vi "PH_Beamline.ProcCases.vi"(0 "i ref in":refnum<vi>, 1 "selector":string, 2 "Data":T1, 3 "call cluster":T2={"Object"="", "Selector"="", "CallType"=enum."synchronous", "Async Object"="", "Async Selector"="", "Data Descriptor"="", "Data"=[], "Error #"=0, "Expire"=0}, 5 "error in (no error)":errorcluster) -> (14 "i ref out":refnum<vi>, 17 "answer cluster":T2={"Object"="", "Selector"="", "CallType"=enum."synchronous", "Async Object"="", "Async Selector"="", "Data Descriptor"="", "Data"=[], "Error #"=0, "Expire"=0}, 19 "error out":errorcluster)   [LabVIEW 2014, in "PH_Beamline.lvlib"]
doc: "This method is called by a process from within the default case in the event loop. The methods of a class that are linked to events will be called from THIS method. Add your code here."
uses:
  PH_Beamline.lvlib
  CS_Core/CSSystem/CoreDefs/CoreDefs.call_type.ctl
  CS_Core/BaseProcess/BaseProcess.descriptor string definition.ctl
  CS_Core/CSSystem/CoreDefs/CoreDefs.rawDataType.ctl
  PH_Beamline_Chief/PH_Beamline_Chief.Settings.ctl
  PH_Basics/PH_StatusHandler/PH_StatusHandler.Status.ctl
  CS_Core/CSSystem/CoreLib/CoreLib.string 2 byte array.vi
  CS_Core/BaseProcess/BaseProcess.lvlib
  PH_Basics/PH_Common/PH_Common.lvlib
  CS_Core/CAEObj/CAEObj.lvlib
  CS_Core/CSSystem/CoreLib/CoreLib.lvlib
  PH_Basics/PH_StatusHandler/PH_StatusHandler.lvlib
  PH_BL-Master/PH_BL-Master.lvlib
  PH_Beamline_Chief/PH_Beamline_Chief.lvlib
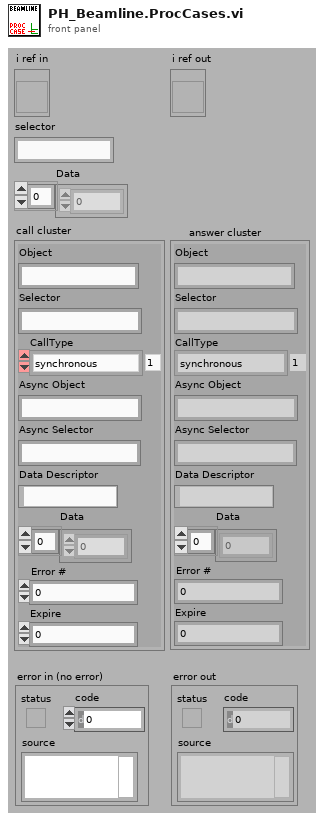
[diagram p1: front panel]
types:
  T1 = typedef "CoreDefs.rawDataType.ctl" = i8[]
  T2 = typedef "CoreDefs.call_type.ctl" = cluster{"Object":string, "Selector":string, "CallType":enum16{"simple", "synchronous", "asynchronous"}, "Async Object":string, "Async Selector":string, "Data Descriptor":T3, "Data":T1, "Error #":i32, "Expire":u32}
  T3 = typedef "BaseProcess.lvlib/BaseProcess.descriptor string definition.ctl" = string
  T4 = typedef "PH_Beamline_Chief.lvlib/PH_Beamline_Chief.Settings.ctl" = cluster{"PA Doublepass Mode":bool, "Compressor Vaccuum LB not relevant":bool, "Windowshutter TB2 not relevant":bool, "Windowshutter TB3 not relevant":bool}
  T5 = typedef "PH_BL-Master.lvlib/PH_BL-Master.i attribute.ctl" = cluster{"Remote controlled":bool, "Boolean Condition Service Subscriber":refnum<vi>[], "Picture Condition Service Subscriber":refnum<vi>[], "R2S":cluster{"GUI Ref":refnum<vi>, "State":bool}, "Vacua":cluster{"GUI Ref":refnum<vi>, "Limit":dbl, "Curr Value":dbl, "in range":bool}[], "O2 Inspection":cluster{"GUI Ref":refnum<vi>, "Concentration":dbl, "State":T6}[], "Boolean Status Service Subscriber":cluster{"GUI Ref":refnum<vi>, "Status":T6, "no Link?":bool, "Status Subscriber Class":T7}[], "Picture Status Service Subscriber":cluster{"GUI Ref":refnum<vi>, "Status":T6, "no Link?":bool, "Status Subscriber Class":T7}[], "6P 4Q Service Subscriber":cluster{"GUI Ref":refnum<vi>, "Selector":T8, "no Link?":bool}[], "Index of latest 6P 4Q changing Instance":i32, "Index of latest Picture Status changing Instance":i32, "Index of latest Boolean Status changing Instance":i32, "Vision ID on same Node":string, "Start Phase over?":bool, "GUI Ref Delete":refnum<vi>}
  T6 = typedef "PH_StatusHandler.lvlib/PH_StatusHandler.Status.ctl" = i16
  T7 = typedef "PH_BL-Master.lvlib/PH_BL-Master.Status Subscriber Class.ctl" = enum16{"unknown", "Switch", "BB", "6P Switch", "Switch GUI", "Switch and 6P State", "Force Sensor"}
  T8 = typedef "PH_4_Pos_Selector.lvlib/PH_4_Pos_Selector.Position Selector.ctl" = u16
  T9 = typedef "PH_Beamline.lvlib/PH_Beamline.i attribute.ctl" = cluster{"GUI Refs":cluster{"PA ok":refnum<vi>, "MA ok":refnum<vi>, "fs FE ok":refnum<vi>, "ns FE ok":refnum<vi>, "PA ED ok":refnum<vi>, "MAS ok":refnum<vi>, "Booster ok":refnum<vi>, "Mirrortower ok":refnum<vi>, "In.-Box ok":refnum<vi>, "Compressor ok":refnum<vi>, "Experiment LB ok":refnum<vi>, "Experiment LL ok":refnum<vi>, "PHELIX_Beckhoff_Watchdog":refnum<vi>, "Shutters closed":refnum<vi>, "uOPA ok":refnum<vi>, "Vacuum no shotcond Comp LB":refnum<vi>}, "Refs BL MA":refnum<vi>[], "Refs BL MA-IB":refnum<vi>[], "Refs BL fs":refnum<vi>[], "Refs BL PA ED":refnum<vi>[], "Refs BL MAS":refnum<vi>[], "Refs BL Boo":refnum<vi>[], "Refs BL ns":refnum<vi>[], "Refs BL Mirrortower":refnum<vi>[], "Refs BL Compressor":refnum<vi>[], "Refs BL Exp LB":refnum<vi>[], "Radiation Safety":cluster{"Exp Laserbay":cluster{"Ref Op Mode":refnum<vi>, "Ref Laserbay evacuated":refnum<vi>, "Tagname LB evacuated":string, "Shot Mode":T10, "Laserbay evacuated?":i32, "Tagname HV room locked":string, "HV room locked?":i32, "Ref HV room locked":refnum<vi>, "Tagname bridged?":string, "Ref Bridge":refnum<vi>, "I<1E18W/cm²":bool}, "Exp Laserlab":cluster{"Ref Op Mode":refnum<vi>, "Ref Laserlab evacuated":refnum<vi>, "Tagname LL evacuated":string, "Shot Mode":T10, "Laserlab evacuated?":i32, "Tagname bridged?":string, "Ref Bridge":refnum<vi>, "I<1E18W/cm²":bool}}, "Refs BL LL":refnum<vi>[], "PP Igni Heating GUI Refs":refnum<vi>[], "PP Igni Heating Tagnames ":string[], "Refs BL PA":cluster{"undelayed Line before Shutter":refnum<vi>[], "undelayed Line after Shutter":refnum<vi>[], "before Bypass":refnum<vi>[], "delayed Line before Shutter":refnum<vi>[], "delayed Line after Shutter":refnum<vi>[], "before Shutter Input":refnum<vi>[], "after Shutter Input":refnum<vi>[], "Bypass":refnum<vi>[], "before Shutter Exit":refnum<vi>[], "after Shutter Exit":refnum<vi>[], "to MA":refnum<vi>[], "to Lab":refnum<vi>[]}, "BL":cluster{"YLF_BL_Status":i32, "fs_BL_Status":i32, "fs_YLF_BL_Status":i32, "ns_BL_Status":i32, "PA_Input_BL_Status":i32, "PA_UnDelay_BL_Status":i32, "PA_Delay_BL_Status":i32, "PA_BL_Status":i32, "PA_Bypass_BL_Status":i32, "PA_Exit_BL_Status":i32, "PA_LL_BL_Status":i32, "LL_BL_Status":i32, "PA_MA_BL_Status":i32, "MA_Exit_BL_Status":i32, "MA_Z6_BL_Status":i32, "Z6_BL_Status":i32, "MA_LB_BL_Status":i32, "LB_TB2_BL_Status":i32, "PA_before_Bypass_BL_Status":i32, "LB_TB3_BL_Status":i32}, "State Subsystems":cluster{"PA":bool, "MA":bool, "ns FE":bool, "fs FE":bool, "PA ED":bool, "In.-Box":bool, "MAS":bool, "Booster":bool, "Mirrortower":bool, "Compressor":bool, "Experiment LB":bool, "Experiment LL":bool, "uOPA":bool}, "Status Subscriber Information":T11, "Refs BL uOPA":refnum<vi>[], "PA_Input_2_Beam_6PWpGUI not linked?":bool, "PA_Input_Delay_6PGUI not linked?":bool, "Settings":T4}
  T10 = typedef "PH_Beamline.lvlib/PH_Beamline.Operation Mode.ctl" = i32
  T11 = typedef "PH_Beamline.lvlib/PH_Beamline.Status Subscriber Information.ctl" = cluster{"fs Swich YLF":T12, "fs Exit Shutter":T12, "ns Exit Shutter":T12, "PA Input Shutter":T12, "PA PC WP":T12, "PA PC WP 2":T12, "PA Bypass In":T12, "PA Bypass Out":T12, "PA CH 1":T12, "PA delayed":T12, "PA non delayed":T12, "PA Exit Shutter":T12, "PA Switch Lab":T12, "PA Bridge CH Input MA":T12, "MA Diffusor IB":T12, "MA IB Ready":T12, "MA CH 1":T12, "MA CH 2":T12, "MA CH 3":T12, "MA CH 4":T12, "MA Shutter Align Cam":T12, "MA Position MM5":T12, "Calorimeter Switch":T12, "BL Z6 CH 9":T12, "BL Z6 Beamdump":T12, "BL Z6 Shutter":T12, "COS Sensitivity Switch":T12, "Exp LB Shutter":T12, "Exp LB TB 2":T12, "Exp LB TB 3":T12, "PA LL Input CH":T12, "PA LL Output CH":T12, "LL Comp Input Shutter":T12, "LL Comp Output Shutter":T12, "LL Comp FF Shutter":T12, "Exp LL Shutter":T12, "MA IM In IB":T12, "MA IM Out IB":T12, "MA DB In IB":T12, "MA DB Out IB":T12, "Exp LB Shutter Interlock":T12, "Exp LL Shutter Interlock":T12, "MM1 Force Sensor":T12}
  T12 = typedef "PH_BL-Master.lvlib/PH_BL-Master.Status Subscriber Information.ctl" = cluster{"Index of element":i32, "Attributeset":T13}
  T13 = typedef "PH_BL-Master.lvlib/PH_BL-Master.Attribute Set.ctl" = enum16{"Boolean Status Service Subscriber", "Picture Status Service Subscriber"}
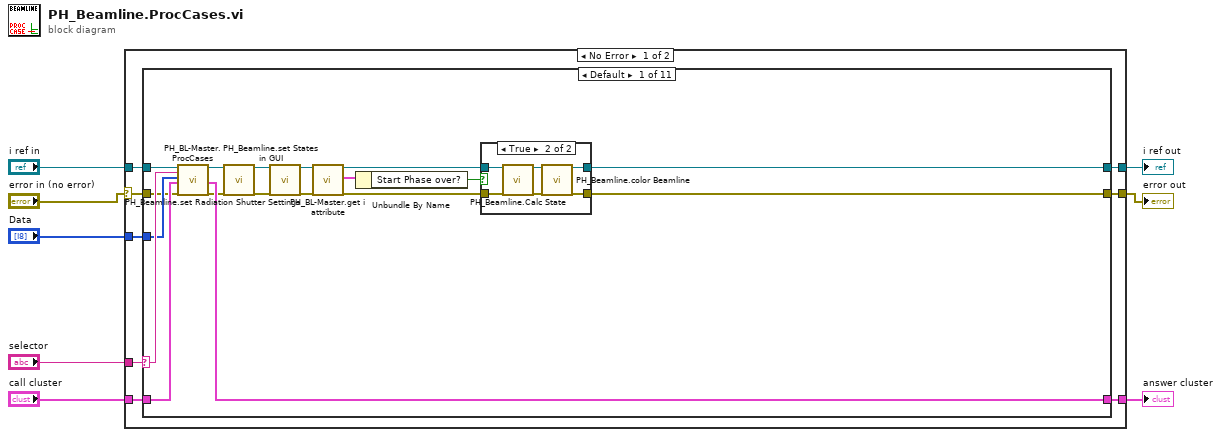
[diagram p0: block diagram]
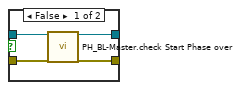
[diagram p2: hidden frame]
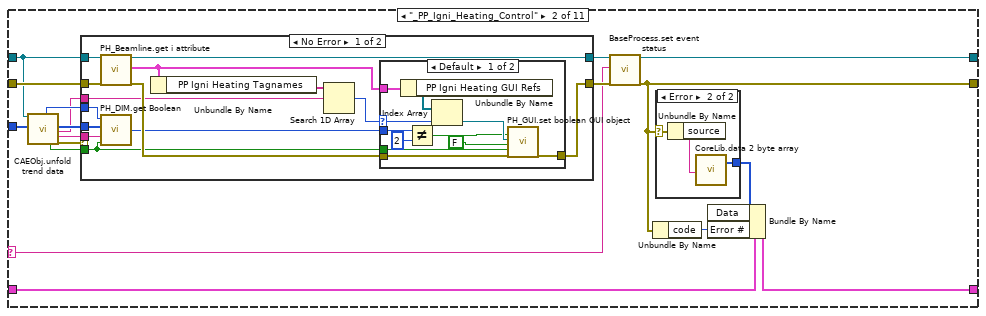
[diagram p3: hidden frame]
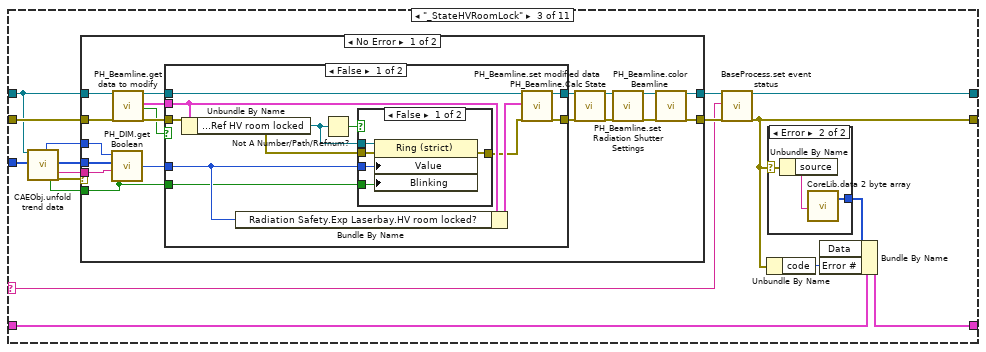
[diagram p7: hidden frame]
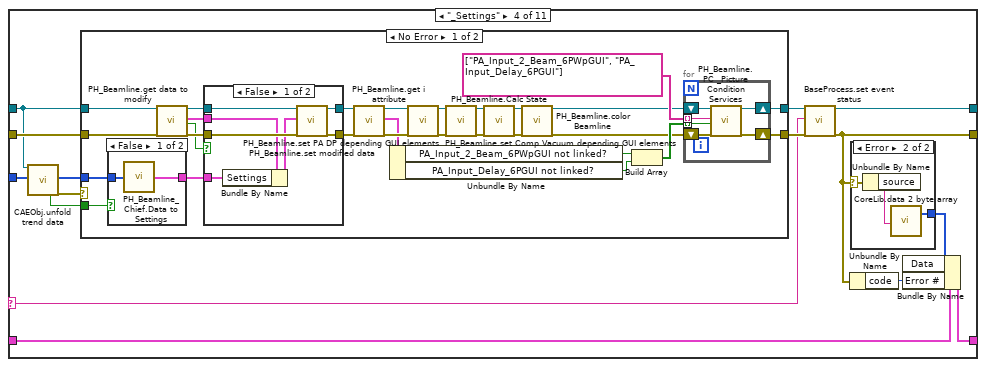
[diagram p12: hidden frame]
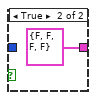
[diagram p14: hidden frame]
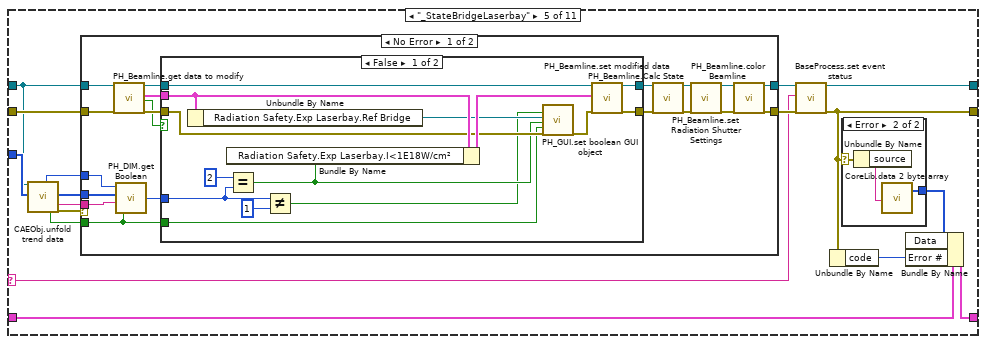
[diagram p17: hidden frame]
diagram:
  n1 = case shown="No Error" "error in (no error)" {
    selector: "error in (no error)" -> [w9 w487]
    tunnel: "selector" -> [w16 _]
    tunnel: [w15 w486] -> w7
    tunnel: "call cluster" -> [w14 w486]
    tunnel: "i ref in" -> [w13 w488]
    tunnel: [w12 w488] -> w4
    tunnel: [w11 w487] -> w3
    tunnel: "Data" -> [w10 _]
    frame No Error {
      n2 = case shown="Default" w16 {
        selector: w16 -> [w32 w47 w96 w156 w222 w279 w338 w371 w409 w445 w479]
        tunnel: w13 -> [w19 w60 w108 w166 w234 w291 w347 w383 w421 w454 w473]
        tunnel: [w31 w48 w97 w157 w223 w280 w339 w372 w410 w448 w478] -> w12
        tunnel: w14 -> [w33 w46 w95 w155 w221 w278 w337 w370 w408 w446 w476]
        tunnel: [w34 w45 w94 w154 w220 w277 w336 w369 w407 w444 w475] -> w15
        tunnel: w9 -> [w20 w62 w110 w168 w236 w293 w349 w385 w423 w457 w474]
        tunnel: [w30 w49 w98 w158 w224 w281 w340 w373 w411 w447 w477] -> w11
        tunnel: w10 -> [w29 w61 w109 w167 w235 w292 w348 w384 w422 w456 _]
        frame Default {
          n3 = call "PH_BL-Master.ProcCases.vi"("i ref in"=w19, "selector"=w32, "Data"=w29, "call cluster"=w33, "error in (no error)"=w20) -> ("i ref out"=w17:refnum<vi>, "answer cluster"=w34:T2, "error out"=w18:errorcluster)  [unwired: 12 in]
          n4 = call "PH_Beamline.set States in GUI.vi"("i ref in"=w17, "error in"=w18) -> ("i ref out"=w21:refnum<vi>, "error out"=w22:errorcluster)  [unwired: 16 in]
          n5 = call "PH_Beamline.set Radiation Shutter Settings.vi"("i ref in"=w21, "error in"=w22) -> ("i ref out"=w26:refnum<vi>, "error out"=w28:errorcluster)  [unwired: 16 in]
          n6 = call "PH_BL-Master.get i attribute.vi"("i ref in"=w26, "error in (no error)"=w28) -> ("i ref out"=w25:refnum<vi>, "i attribute"=w24:T5, "error out"=w27:errorcluster)  [unwired: 15 in]
          n7 = Unbundle By Name(w24) -> ("Start Phase over?"=w23:bool)
          n8 = case shown="True" w23 {
            tunnel: [w37 w44] -> w31
            tunnel: [w35 w43] -> w30
            tunnel: w27 -> [w36 w40]
            tunnel: w25 -> [w38 w39]
            frame False {
              n9 = call "PH_BL-Master.check Start Phase over.vi"("VI in"=w38, "error in (no error)"=w36) -> ("VI out"=w37:refnum<vi>, "error out"=w35:errorcluster)  [unwired: 16 in]
            }
            frame True {
              n10 = call "PH_Beamline.Calc State.vi"("i ref in"=w39, "error in (no error)"=w40) -> ("i ref out"=w42:refnum<vi>, "error out"=w41:errorcluster)  [unwired: 16 in]
              n11 = call "PH_Beamline.color Beamline.vi"("i ref in"=w42, "error in (no error)"=w41) -> ("i ref out"=w44:refnum<vi>, "error out"=w43:errorcluster)  [unwired: 16 in]
            }
          }
        }
        frame "_PP_Igni_Heating_Control" {
          n12 = call "CAEObj.unfold trend data.vi"("i ref in"=w60, "raw trend data"=w61) -> ("quality"=w58:i32, "no link"=w57:bool, "data"=w56:i8[], "serviceName"=w54:string, "typeDescriptor"=w55:string, "error out"=w59:errorcluster)  [unwired: 9 in, 3 out]
          n13 = case shown="No Error" w59 {
            tunnel: [w70 w93] -> w51
            tunnel: w60 -> [w74 w93]
            tunnel: w62 -> [w73 w92]
            tunnel: [w69 w92] -> w50
            tunnel: w58 -> [w77 _]
            tunnel: w57 -> [w66 _]
            tunnel: w56 -> [w76 _]
            tunnel: w55 -> [w75 _]
            tunnel: w54 -> [w78 _]
            frame No Error {
              n14 = call "PH_Beamline.get i attribute.vi"("i ref in"=w74, "error in (no error)"=w73) -> ("i ref out"=w70:refnum<vi>, "i attribute"=w68:T9, "error out"=w79:errorcluster)  [unwired: 15 in]
              n15 = call "PH_DIM.get Boolean.vi"("no link"=w66, "typeDescriptor"=w75, "data"=w76, "quality"=w77) -> ("Value"=w67:i32)
              n16 = Unbundle By Name(w68) -> ("PP Igni Heating Tagnames"=w71:string[])
              n17 = Search 1D Array(1D array=w71, element=w78) -> (index of element=w72:i32)  [unwired: 1 in]
              n18 = case shown="Default" w72 {
                selector: w72 -> [w86 _]
                tunnel: w68 -> [w88 _]
                tunnel: w79 -> [w90 w91]
                tunnel: [w89 w91] -> w69
                tunnel: w67 -> [w84 _]
                tunnel: w66 -> [w81 _]
                frame Default {
                  n19 = Unbundle By Name(w88) -> ("PP Igni Heating GUI Refs"=w87:refnum<vi>[])
                  n20 = Not Equal?(x=w84, y=2) -> (x != y?=w82:bool)
                  n21 = Index Array(array=w87, index=w86) -> (element=w85:refnum<vi>)
                  n22 = call "PH_GUI.set boolean GUI object.vi"("Visible (true)"=w82, "Boolean Knob GUI Ref"=w85, "Value"=FALSE, "Blinking? (false)"=w81, "error in (no error)"=w90) -> ("error out"=w89:errorcluster)  [unwired: 14 in]
                }
                frame -1 {
                }
              }
            }
            frame Error {
            }
          }
          n23 = call "BaseProcess.set event status.vi"("i ref in"=w51, "EventStatus"=w47, "error in (no error)"=w50) -> ("i ref out"=w48:refnum<vi>, "error out"=w49:errorcluster)  [unwired: 14 in, 1 out]
          n24 = Unbundle By Name(w49) -> ("code"=w53:i32)
          n25 = case shown="Error" w49 {
            selector: w49 -> [_ w65]
            tunnel: [_ w63] -> w52
            frame No Error {
            }
            frame Error {
              n26 = Unbundle By Name(w65) -> ("source"=w64:string)
              n27 = call-poly "CoreLib.data 2 byte array.vi"("string"=w64) -> ("byteArray out"=w63:T1)  [unwired: 18 in]
            }
          }
          n28 = Bundle By Name(cluster=w46, "Data"=w52, "Error #"=w53) -> (w45:T2)
        }
        frame "_StateHVRoomLock" {
          n29 = call "CAEObj.unfold trend data.vi"("i ref in"=w108, "raw trend data"=w109) -> ("quality"=w106:i32, "no link"=w105:bool, "data"=w104:i8[], "typeDescriptor"=w103:string, "error out"=w107:errorcluster)  [unwired: 9 in, 4 out]
          n30 = case shown="No Error" w107 {
            tunnel: [w119 w153] -> w100
            tunnel: w108 -> [w129 w153]
            tunnel: w110 -> [w128 w152]
            tunnel: [w115 w152] -> w99
            tunnel: w106 -> [w132 _]
            tunnel: w105 -> [w124 _]
            tunnel: w104 -> [w131 _]
            tunnel: w103 -> [w130 _]
            frame No Error {
              n31 = call "PH_DIM.get Boolean.vi"("no link"=w124, "typeDescriptor"=w130, "data"=w131, "quality"=w132) -> ("Value"=w125:i32)
              n32 = call "PH_Beamline.get data to modify.vi"("i ref in"=w129, "error in (no error)"=w128) -> ("i ref out"=w127:refnum<vi>, "i attribute"=w126:T9, "timed out"=w122:bool, "error out"=w123:errorcluster)  [unwired: 14 in]
              n33 = case shown="False" w122 {
                tunnel: w127 -> [w143 w151]
                tunnel: [w142 w151] -> w118
                tunnel: [w141 w150] -> w114
                tunnel: w126 -> [w140 _]
                tunnel: w125 -> [w137 _]
                tunnel: w124 -> [w136 _]
                tunnel: w123 -> [w134 w150]
                frame False {
                  n34 = Unbundle By Name(w140) -> ("Radiation Safety.Exp Laserbay.Ref HV room locked"=w135:refnum<vi>)
                  n35 = Bundle By Name(cluster=w140, "Radiation Safety.Exp Laserbay.HV room locked?"=w137) -> (w139:T9)
                  n36 = Not A Number/Path/Refnum?(number/path/refnum=w135) -> (NaN/Path/Refnum?=w138:bool)
                  n37 = case shown="False" w138 {
                    tunnel: w134 -> [w148 w149]
                    tunnel: [w147 w149] -> w133
                    tunnel: w135 -> [w146 _]
                    tunnel: w137 -> [w145 _]
                    tunnel: w136 -> [w144 _]
                    frame False {
                      n38 = property class="Ring (strict)"(reference=w146, error in=w148, "Value"=w145, "Blinking"=w144) -> (error out=w147:errorcluster)  [unwired: 1 out]
                    }
                    frame True {
                    }
                  }
                  n39 = call "PH_Beamline.set modified data.vi"("i ref in"=w143, "i attribute"=w139, "error in (no error)"=w133) -> ("i ref out"=w142:refnum<vi>, "error out"=w141:errorcluster)  [unwired: 15 in]
                }
                frame True {
                }
              }
              n40 = call "PH_Beamline.Calc State.vi"("i ref in"=w118, "error in (no error)"=w114) -> ("i ref out"=w121:refnum<vi>, "error out"=w117:errorcluster)  [unwired: 16 in]
              n41 = call "PH_Beamline.set Radiation Shutter Settings.vi"("i ref in"=w121, "error in"=w117) -> ("i ref out"=w120:refnum<vi>, "error out"=w116:errorcluster)  [unwired: 16 in]
              n42 = call "PH_Beamline.color Beamline.vi"("i ref in"=w120, "error in (no error)"=w116) -> ("i ref out"=w119:refnum<vi>, "error out"=w115:errorcluster)  [unwired: 16 in]
            }
            frame Error {
            }
          }
          n43 = call "BaseProcess.set event status.vi"("i ref in"=w100, "EventStatus"=w96, "error in (no error)"=w99) -> ("i ref out"=w97:refnum<vi>, "error out"=w98:errorcluster)  [unwired: 14 in, 1 out]
          n44 = Unbundle By Name(w98) -> ("code"=w102:i32)
          n45 = case shown="Error" w98 {
            selector: w98 -> [_ w113]
            tunnel: [_ w111] -> w101
            frame No Error {
            }
            frame Error {
              n46 = Unbundle By Name(w113) -> ("source"=w112:string)
              n47 = call-poly "CoreLib.data 2 byte array.vi"("string"=w112) -> ("byteArray out"=w111:T1)  [unwired: 18 in]
            }
          }
          n48 = Bundle By Name(cluster=w95, "Data"=w101, "Error #"=w102) -> (w94:T2)
        }
        frame "_Settings" {
          n49 = call "CAEObj.unfold trend data.vi"("i ref in"=w166, "raw trend data"=w167) -> ("no link"=w164:bool, "data"=w163:i8[], "error out"=w165:errorcluster)  [unwired: 9 in, 6 out]
          n50 = case shown="No Error" w165 {
            tunnel: [w173 w219] -> w160
            tunnel: w166 -> [w199 w219]
            tunnel: w168 -> [w198 w218]
            tunnel: [w172 w218] -> w159
            tunnel: w164 -> [w192 _]
            tunnel: w163 -> [w193 _]
            frame No Error {
              n51 = case shown="False" w192 {
                tunnel: w193 -> [w207 _]
                tunnel: [w206 T4 {"PA Doublepass Mode"=FALSE, "Compressor Vaccuum LB not relevant"=FALSE, "Windowshutter TB2 not relevant"=FALSE, "Windowshutter TB3 not relevant"=FALSE} ("Settings")] -> w191
                frame False {
                  n52 = call "PH_Beamline_Chief.Data to Settings.vi"("data"=w207) -> ("Settings"=w206:T4)
                }
                frame True {
                }
              }
              n53 = call "PH_Beamline.get data to modify.vi"("i ref in"=w199, "error in (no error)"=w198) -> ("i ref out"=w197:refnum<vi>, "i attribute"=w196:T9, "timed out"=w194:bool, "error out"=w195:errorcluster)  [unwired: 14 in]
              n54 = case shown="False" w194 {
                tunnel: w197 -> [w215 w217]
                tunnel: [w210 w217] -> w182
                tunnel: [w211 w216] -> w184
                tunnel: w196 -> [w212 _]
                tunnel: w195 -> [w214 w216]
                tunnel: w191 -> [w209 _]
                frame False {
                  n55 = Bundle By Name(cluster=w212, "Settings"=w209) -> (w213:T9)
                  n56 = call "PH_Beamline.set modified data.vi"("i ref in"=w215, "i attribute"=w213, "error in (no error)"=w214) -> ("i ref out"=w210:refnum<vi>, "error out"=w211:errorcluster)  [unwired: 15 in]
                }
                frame True {
                }
              }
              n57 = call "PH_Beamline.get i attribute.vi"("i ref in"=w182, "error in (no error)"=w184) -> ("i ref out"=w181:refnum<vi>, "i attribute"=w176:T9, "error out"=w183:errorcluster)  [unwired: 15 in]
              n58 = Unbundle By Name(w176) -> ("PA_Input_2_Beam_6PWpGUI not linked?"=w177:bool, "PA_Input_Delay_6PGUI not linked?"=w178:bool)
              n59 = call "PH_Beamline.set PA DP depending GUI elements.vi"("VI in"=w181, "error in (no error)"=w183) -> ("VI out"=w190:refnum<vi>, "error out"=w189:errorcluster)  [unwired: 16 in]
              n60 = call "PH_Beamline.set Comp Vacuum depending GUI elements.vi"("VI in"=w190, "error in (no error)"=w189) -> ("VI out"=w188:refnum<vi>, "error out"=w186:errorcluster)  [unwired: 16 in]
              n61 = call "PH_Beamline.Calc State.vi"("i ref in"=w188, "error in (no error)"=w186) -> ("i ref out"=w187:refnum<vi>, "error out"=w185:errorcluster)  [unwired: 16 in]
              n62 = call "PH_Beamline.color Beamline.vi"("i ref in"=w187, "error in (no error)"=w185) -> ("i ref out"=w175:refnum<vi>, "error out"=w174:errorcluster)  [unwired: 16 in]
              n63 = Build Array(w177, w178) -> (w179:bool[])
              n64 = for {
                tunnel: w179 -> [w201] mode=indexing
                tunnel: string[] ["PA_Input_2_Beam_6PWpGUI", "PA_Input_Delay_6PGUI"] -> [w200] mode=indexing
                shift-right: [w204] -> w173
                shift-left: w175 -> [w205]
                shift-right: [w202] -> w172
                shift-left: w174 -> [w203]
                n65 = call "PH_Beamline.PC _Picture Condition Services.vi"("i ref in"=w205, "Instancename"=w200, "No Link?"=w201, "error IO"=w203) -> ("i ref out"=w204:refnum<vi>, "error out"=w202:errorcluster)  [unwired: 14 in]
              }
            }
            frame Error {
            }
          }
          n66 = call "BaseProcess.set event status.vi"("i ref in"=w160, "EventStatus"=w156, "error in (no error)"=w159) -> ("i ref out"=w157:refnum<vi>, "error out"=w158:errorcluster)  [unwired: 14 in, 1 out]
          n67 = Unbundle By Name(w158) -> ("code"=w162:i32)
          n68 = case shown="Error" w158 {
            selector: w158 -> [_ w171]
            tunnel: [_ w169] -> w161
            frame No Error {
            }
            frame Error {
              n69 = Unbundle By Name(w171) -> ("source"=w170:string)
              n70 = call-poly "CoreLib.data 2 byte array.vi"("string"=w170) -> ("byteArray out"=w169:T1)  [unwired: 18 in]
            }
          }
          n71 = Bundle By Name(cluster=w155, "Data"=w161, "Error #"=w162) -> (w154:T2)
        }
        frame "_StateBridgeLaserbay" {
          n72 = call "CAEObj.unfold trend data.vi"("i ref in"=w234, "raw trend data"=w235) -> ("quality"=w232:i32, "no link"=w231:bool, "data"=w230:i8[], "typeDescriptor"=w229:string, "error out"=w233:errorcluster)  [unwired: 9 in, 4 out]
          n73 = case shown="No Error" w233 {
            tunnel: [w245 w276] -> w226
            tunnel: w234 -> [w255 w276]
            tunnel: w236 -> [w254 w275]
            tunnel: [w241 w275] -> w225
            tunnel: w232 -> [w258 _]
            tunnel: w231 -> [w250 _]
            tunnel: w230 -> [w257 _]
            tunnel: w229 -> [w256 _]
            frame No Error {
              n74 = call "PH_Beamline.get data to modify.vi"("i ref in"=w255, "error in (no error)"=w254) -> ("i ref out"=w253:refnum<vi>, "i attribute"=w252:T9, "timed out"=w248:bool, "error out"=w249:errorcluster)  [unwired: 14 in]
              n75 = call "PH_DIM.get Boolean.vi"("no link"=w250, "typeDescriptor"=w256, "data"=w257, "quality"=w258) -> ("Value"=w251:i32)
              n76 = case shown="False" w248 {
                tunnel: w253 -> [w272 w274]
                tunnel: [w271 w274] -> w244
                tunnel: [w270 w273] -> w240
                tunnel: w252 -> [w269 _]
                tunnel: w251 -> [w261 _]
                tunnel: w250 -> [w264 _]
                tunnel: w249 -> [w267 w273]
                frame False {
                  n77 = Unbundle By Name(w269) -> ("Radiation Safety.Exp Laserbay.Ref Bridge"=w265:refnum<vi>)
                  n78 = Equal?(x=2, y=w261) -> (x = y?=w262:bool)
                  n79 = Bundle By Name(cluster=w269, "Radiation Safety.Exp Laserbay.I<1E18W/cm²"=w262) -> (w268:T9)
                  n80 = Not Equal?(x=w261, y=1) -> (x != y?=w259:bool)
                  n81 = call "PH_GUI.set boolean GUI object.vi"("Visible (true)"=w259, "Boolean Knob GUI Ref"=w265, "Value"=w262, "Blinking? (false)"=w264, "error in (no error)"=w267) -> ("error out"=w266:errorcluster)  [unwired: 14 in]
                  n82 = call "PH_Beamline.set modified data.vi"("i ref in"=w272, "i attribute"=w268, "error in (no error)"=w266) -> ("i ref out"=w271:refnum<vi>, "error out"=w270:errorcluster)  [unwired: 15 in]
                }
                frame True {
                }
              }
              n83 = call "PH_Beamline.Calc State.vi"("i ref in"=w244, "error in (no error)"=w240) -> ("i ref out"=w247:refnum<vi>, "error out"=w243:errorcluster)  [unwired: 16 in]
              n84 = call "PH_Beamline.set Radiation Shutter Settings.vi"("i ref in"=w247, "error in"=w243) -> ("i ref out"=w246:refnum<vi>, "error out"=w242:errorcluster)  [unwired: 16 in]
              n85 = call "PH_Beamline.color Beamline.vi"("i ref in"=w246, "error in (no error)"=w242) -> ("i ref out"=w245:refnum<vi>, "error out"=w241:errorcluster)  [unwired: 16 in]
            }
            frame Error {
            }
          }
          n86 = call "BaseProcess.set event status.vi"("i ref in"=w226, "EventStatus"=w222, "error in (no error)"=w225) -> ("i ref out"=w223:refnum<vi>, "error out"=w224:errorcluster)  [unwired: 14 in, 1 out]
          n87 = Unbundle By Name(w224) -> ("code"=w228:i32)
          n88 = case shown="Error" w224 {
            selector: w224 -> [_ w239]
            tunnel: [_ w237] -> w227
            frame No Error {
            }
            frame Error {
              n89 = Unbundle By Name(w239) -> ("source"=w238:string)
              n90 = call-poly "CoreLib.data 2 byte array.vi"("string"=w238) -> ("byteArray out"=w237:T1)  [unwired: 18 in]
            }
          }
          n91 = Bundle By Name(cluster=w221, "Data"=w227, "Error #"=w228) -> (w220:T2)
        }
        frame "_StateBridgeLaserlab" {
          n92 = call "CAEObj.unfold trend data.vi"("i ref in"=w291, "raw trend data"=w292) -> ("quality"=w289:i32, "no link"=w288:bool, "data"=w287:i8[], "typeDescriptor"=w286:string, "error out"=w290:errorcluster)  [unwired: 9 in, 4 out]
          n93 = case shown="No Error" w290 {
            tunnel: [w302 w333] -> w283
            tunnel: w291 -> [w312 w333]
            tunnel: w293 -> [w311 w332]
            tunnel: [w298 w332] -> w282
            tunnel: w289 -> [w315 _]
            tunnel: w288 -> [w307 _]
            tunnel: w287 -> [w314 _]
            tunnel: w286 -> [w313 _]
            frame No Error {
              n94 = call "PH_Beamline.get data to modify.vi"("i ref in"=w312, "error in (no error)"=w311) -> ("i ref out"=w310:refnum<vi>, "i attribute"=w309:T9, "timed out"=w305:bool, "error out"=w306:errorcluster)  [unwired: 14 in]
              n95 = call "PH_DIM.get Boolean.vi"("no link"=w307, "typeDescriptor"=w313, "data"=w314, "quality"=w315) -> ("Value"=w308:i32)
              n96 = case shown="False" w305 {
                tunnel: w310 -> [w329 w331]
                tunnel: [w328 w331] -> w301
                tunnel: [w327 w330] -> w297
                tunnel: w309 -> [w326 _]
                tunnel: w308 -> [w318 _]
                tunnel: w307 -> [w321 _]
                tunnel: w306 -> [w324 w330]
                frame False {
                  n97 = Unbundle By Name(w326) -> ("Radiation Safety.Exp Laserlab.Ref Bridge"=w322:refnum<vi>)
                  n98 = Equal?(x=2, y=w318) -> (x = y?=w319:bool)
                  n99 = Bundle By Name(cluster=w326, "Radiation Safety.Exp Laserlab.I<1E18W/cm²"=w319) -> (w325:T9)
                  n100 = Not Equal?(x=w318, y=1) -> (x != y?=w316:bool)
                  n101 = call "PH_GUI.set boolean GUI object.vi"("Visible (true)"=w316, "Boolean Knob GUI Ref"=w322, "Value"=w319, "Blinking? (false)"=w321, "error in (no error)"=w324) -> ("error out"=w323:errorcluster)  [unwired: 14 in]
                  n102 = call "PH_Beamline.set modified data.vi"("i ref in"=w329, "i attribute"=w325, "error in (no error)"=w323) -> ("i ref out"=w328:refnum<vi>, "error out"=w327:errorcluster)  [unwired: 15 in]
                }
                frame True {
                }
              }
              n103 = call "PH_Beamline.Calc State.vi"("i ref in"=w301, "error in (no error)"=w297) -> ("i ref out"=w304:refnum<vi>, "error out"=w300:errorcluster)  [unwired: 16 in]
              n104 = call "PH_Beamline.set Radiation Shutter Settings.vi"("i ref in"=w304, "error in"=w300) -> ("i ref out"=w303:refnum<vi>, "error out"=w299:errorcluster)  [unwired: 16 in]
              n105 = call "PH_Beamline.color Beamline.vi"("i ref in"=w303, "error in (no error)"=w299) -> ("i ref out"=w302:refnum<vi>, "error out"=w298:errorcluster)  [unwired: 16 in]
            }
            frame Error {
            }
          }
          n106 = call "BaseProcess.set event status.vi"("i ref in"=w283, "EventStatus"=w279, "error in (no error)"=w282) -> ("i ref out"=w280:refnum<vi>, "error out"=w281:errorcluster)  [unwired: 14 in, 1 out]
          n107 = Unbundle By Name(w281) -> ("code"=w285:i32)
          n108 = case shown="Error" w281 {
            selector: w281 -> [_ w296]
            tunnel: [_ w294] -> w284
            frame No Error {
            }
            frame Error {
              n109 = Unbundle By Name(w296) -> ("source"=w295:string)
              n110 = call-poly "CoreLib.data 2 byte array.vi"("string"=w295) -> ("byteArray out"=w294:T1)  [unwired: 18 in]
            }
          }
          n111 = Bundle By Name(cluster=w278, "Data"=w284, "Error #"=w285) -> (w277:T2)
        }
        frame "_PHELIX_Beckhoff_Watchdog" {
          n112 = call "CAEObj.unfold trend data.vi"("i ref in"=w347, "raw trend data"=w348) -> ("no link"=w345:bool, "data"=w334:i8[], "typeDescriptor"=w335:string, "error out"=w346:errorcluster)  [unwired: 9 in, 5 out]
          n113 = case shown="No Error" w346 {
            tunnel: [w363 w368] -> w342
            tunnel: w347 -> [w365 w368]
            tunnel: w349 -> [w364 w367]
            tunnel: [w362 w367] -> w341
            tunnel: w345 -> [w355 _]
            tunnel: w335 -> [w357 _]
            tunnel: w334 -> [w356 _]
            frame No Error {
              w353 = T6 2 items=["no info", "off/false/out", "on/true/in", "Failure", "Alarm", "Status 1", "Status 2", "Status 3"] ("Status")
              n114 = call "PH_StatusHandler.get Status DIM Service.vi"("no link"=w355, "typeDescriptor"=w357, "data"=w356) -> ("Status"=w354:T6)  [unwired: 1 in]
              n115 = call "PH_Beamline.get i attribute.vi"("i ref in"=w365, "error in (no error)"=w364) -> ("i ref out"=w363:refnum<vi>, "i attribute"=w361:T9, "error out"=w366:errorcluster)  [unwired: 15 in]
              n116 = Unbundle By Name(w361) -> ("GUI Refs.PHELIX_Beckhoff_Watchdog"=w358:refnum<vi>)
              n117 = Not Equal?(x=w354, y=w353) -> (x != y?=w360:bool)
              n118 = call "PH_GUI.set boolean GUI object.vi"("Visible (true)"=w360, "Boolean Knob GUI Ref"=w358, "Value"=TRUE, "Blinking? (false)"=w355, "error in (no error)"=w366) -> ("error out"=w362:errorcluster)  [unwired: 14 in]
            }
            frame Error {
            }
          }
          n119 = call "BaseProcess.set event status.vi"("i ref in"=w342, "EventStatus"=w338, "error in (no error)"=w341) -> ("i ref out"=w339:refnum<vi>, "error out"=w340:errorcluster)  [unwired: 14 in, 1 out]
          n120 = Unbundle By Name(w340) -> ("code"=w344:i32)
          n121 = case shown="Error" w340 {
            selector: w340 -> [_ w352]
            tunnel: [_ w350] -> w343
            frame No Error {
            }
            frame Error {
              n122 = Unbundle By Name(w352) -> ("source"=w351:string)
              n123 = call-poly "CoreLib.data 2 byte array.vi"("string"=w351) -> ("byteArray out"=w350:T1)  [unwired: 18 in]
            }
          }
          n124 = Bundle By Name(cluster=w337, "Data"=w343, "Error #"=w344) -> (w336:T2)
        }
        frame "_Shotmode" {
          n125 = call "CAEObj.unfold trend data.vi"("i ref in"=w383, "raw trend data"=w384) -> ("quality"=w381:i32, "no link"=w380:bool, "data"=w379:i8[], "typeDescriptor"=w378:string, "error out"=w382:errorcluster)  [unwired: 9 in, 4 out]
          n126 = case shown="No Error" w382 {
            tunnel: [w393 w405] -> w375
            tunnel: w383 -> [w390 w405]
            tunnel: w385 -> [w389 w404]
            tunnel: [w394 w404] -> w374
            tunnel: w381 -> [w403 _]
            tunnel: w380 -> [w391 _]
            tunnel: w379 -> [w402 _]
            tunnel: w378 -> [w401 _]
            frame No Error {
              n127 = call "PH_DIM.get Boolean.vi"("no link"=w391, "typeDescriptor"=w401, "data"=w402, "quality"=w403) -> ("Value"=w392:i32)
              n128 = call "PH_Beamline.PC _Shotmode.vi"("i ref in"=w390, "DIM Service Value"=w392, "No link"=w391, "error in"=w389) -> ("i ref out"=w398:refnum<vi>, "error out"=w397:errorcluster)  [unwired: 14 in]
              n129 = call "PH_Beamline.Calc State.vi"("i ref in"=w398, "error in (no error)"=w397) -> ("i ref out"=w400:refnum<vi>, "error out"=w399:errorcluster)  [unwired: 16 in]
              n130 = call "PH_Beamline.color Beamline.vi"("i ref in"=w400, "error in (no error)"=w399) -> ("i ref out"=w396:refnum<vi>, "error out"=w395:errorcluster)  [unwired: 16 in]
              n131 = call "PH_Beamline.set Radiation Shutter Settings.vi"("i ref in"=w396, "error in"=w395) -> ("i ref out"=w393:refnum<vi>, "error out"=w394:errorcluster)  [unwired: 16 in]
            }
            frame Error {
            }
          }
          n132 = call "BaseProcess.set event status.vi"("i ref in"=w375, "EventStatus"=w371, "error in (no error)"=w374) -> ("i ref out"=w372:refnum<vi>, "error out"=w373:errorcluster)  [unwired: 14 in, 1 out]
          n133 = Unbundle By Name(w373) -> ("code"=w377:i32)
          n134 = case shown="Error" w373 {
            selector: w373 -> [_ w388]
            tunnel: [_ w386] -> w376
            frame No Error {
            }
            frame Error {
              n135 = Unbundle By Name(w388) -> ("source"=w387:string)
              n136 = call-poly "CoreLib.data 2 byte array.vi"("string"=w387) -> ("byteArray out"=w386:T1)  [unwired: 18 in]
            }
          }
          n137 = Bundle By Name(cluster=w370, "Data"=w376, "Error #"=w377) -> (w369:T2)
        }
        frame "_EvacuatedState" {
          n138 = call "CAEObj.unfold trend data.vi"("i ref in"=w421, "raw trend data"=w422) -> ("quality"=w419:i32, "no link"=w418:bool, "data"=w417:i8[], "serviceName"=w406:string, "typeDescriptor"=w416:string, "error out"=w420:errorcluster)  [unwired: 9 in, 3 out]
          n139 = case shown="No Error" w420 {
            tunnel: [w436 w442] -> w413
            tunnel: w421 -> [w434 w442]
            tunnel: w423 -> [w433 w441]
            tunnel: [w435 w441] -> w412
            tunnel: w419 -> [w440 _]
            tunnel: w418 -> [w429 _]
            tunnel: w417 -> [w439 _]
            tunnel: w416 -> [w428 _]
            tunnel: w406 -> [w427 _]
            frame No Error {
              n140 = call "PH_DIM.get Boolean.vi"("no link"=w429, "typeDescriptor"=w428, "data"=w439, "quality"=w440) -> ("Value"=w430:i32)
              n141 = call "PH_Beamline.PC _EvacuatedState.vi"("i ref in"=w434, "Value"=w430, "Service Name"=w427, "no link"=w429, "error IO"=w433) -> ("i ref out"=w432:refnum<vi>, "error out"=w431:errorcluster)  [unwired: 13 in]
              n142 = call "PH_Beamline.Calc State.vi"("i ref in"=w432, "error in (no error)"=w431) -> ("i ref out"=w438:refnum<vi>, "error out"=w437:errorcluster)  [unwired: 16 in]
              n143 = call "PH_Beamline.color Beamline.vi"("i ref in"=w438, "error in (no error)"=w437) -> ("i ref out"=w436:refnum<vi>, "error out"=w435:errorcluster)  [unwired: 16 in]
            }
            frame Error {
            }
          }
          n144 = call "BaseProcess.set event status.vi"("i ref in"=w413, "EventStatus"=w409, "error in (no error)"=w412) -> ("i ref out"=w410:refnum<vi>, "error out"=w411:errorcluster)  [unwired: 14 in, 1 out]
          n145 = case shown="Error" w411 {
            selector: w411 -> [_ w426]
            tunnel: [_ w424] -> w414
            frame No Error {
            }
            frame Error {
              n146 = Unbundle By Name(w426) -> ("source"=w425:string)
              n147 = call-poly "CoreLib.data 2 byte array.vi"("string"=w425) -> ("byteArray out"=w424:T1)  [unwired: 18 in]
            }
          }
          n148 = Unbundle By Name(w411) -> ("code"=w415:i32)
          n149 = Bundle By Name(cluster=w408, "Data"=w414, "Error #"=w415) -> (w407:T2)
        }
        frame "_Picture_Condition_Services" {
          n150 = call "CAEObj.unfold trend data.vi"("i ref in"=w454, "raw trend data"=w456) -> ("no link"=w443:bool, "serviceName"=w453:string, "error out"=w455:errorcluster)  [unwired: 9 in, 6 out]
          n151 = case shown="No Error" w455 {
            tunnel: [w468 w470] -> w450
            tunnel: w454 -> [w462 w470]
            tunnel: w457 -> [w467 w469]
            tunnel: [w463 w469] -> w449
            tunnel: w453 -> [w466 _]
            tunnel: w443 -> [w461 _]
            frame No Error {
              n152 = Match Pattern(string=w466, regular expression="_condition") -> (before substring=w464:string)  [unwired: 1 in, 3 out]
              n153 = call "PH_Beamline.PC _Picture Condition Services.vi"("i ref in"=w462, "Instancename"=w464, "No Link?"=w461, "error IO"=w467) -> ("i ref out"=w468:refnum<vi>, "error out"=w463:errorcluster)  [unwired: 14 in]
            }
            frame Error {
            }
          }
          n154 = call "BaseProcess.set event status.vi"("i ref in"=w450, "EventStatus"=w445, "error in (no error)"=w449) -> ("i ref out"=w448:refnum<vi>, "error out"=w447:errorcluster)  [unwired: 14 in, 1 out]
          n155 = case shown="No Error" w447 {
            selector: w447 -> [_ w460]
            tunnel: [_ w458] -> w451
            frame No Error {
            }
            frame Error {
              n156 = Unbundle By Name(w460) -> ("source"=w459:string)
              n157 = call-poly "CoreLib.data 2 byte array.vi"("string"=w459) -> ("byteArray out"=w458:T1)  [unwired: 18 in]
            }
          }
          n158 = Unbundle By Name(w447) -> ("code"=w452:i32)
          n159 = Bundle By Name(cluster=w446, "Data"=w451, "Error #"=w452) -> (w444:T2)
        }
        frame "ClearBL" {
          n160 = call "PH_Beamline.PC Clear beamline.vi"("i ref in"=w473, "error IO"=w474) -> ("i ref out"=w472:refnum<vi>, "error out"=w471:errorcluster)  [unwired: 16 in]
          n161 = call "BaseProcess.set event status.vi"("i ref in"=w472, "EventStatus"=w479, "error in (no error)"=w471) -> ("i ref out"=w478:refnum<vi>, "error out"=w477:errorcluster)  [unwired: 14 in, 1 out]
          n162 = Unbundle By Name(w477) -> ("code"=w481:i32)
          n163 = case shown="Error" w477 {
            selector: w477 -> [_ w485]
            tunnel: [T1 [] ("byteArray out") w483] -> w480
            frame No Error {
            }
            frame Error {
              n164 = Unbundle By Name(w485) -> ("source"=w484:string)
              n165 = call-poly "CoreLib.data 2 byte array.vi"("string"=w484) -> ("byteArray out"=w483:T1)  [unwired: 18 in]
            }
          }
          n166 = Bundle By Name(cluster=w476, "Data"=w480, "Error #"=w481) -> (w475:T2)
        }
      }
    }
    frame Error {
    }
  }
  "answer cluster" <- w7
  "i ref out" <- w4
  "error out" <- w3
